vi "All-Indentify-To-Sort_Lite.vi"(6 "當前位置":i32, 7 "輸出顏色-位置":T1(array[cluster]), 8 "Error In":errorcluster, 11 "HiTechnicColorSensorV2 Ref In":cluster{"I2C Ref Out":T3}) -> (0 "Error Out":errorcluster, 2 "判斷結果":T2, 3 "HiTechnicColorSensorV2 Ref Out":cluster{"I2C Ref Out":T3}, 4 "離家數值":dbl[](array[numeric]), 5 "輸出顏色-位置 2":T1(array[cluster]))   [LabVIEW 2019]
uses:
  <vilib>/myRIO/Instrument Drivers/Onboard IO/I2C/typedefs/I2C Reference.ctl
  <vilib>/myRIO/Common/Instrument Driver Framework/Utilities/typedefs/myRIO Generic Hardware Reference.ctl
  <vilib>/myRIO/Common/Instrument Driver Framework/Utilities/typedefs/Hardware Version Enum.ctl
  <vilib>/myRIO/Common/Instrument Driver Framework/Utilities/typedefs/myRIO v1.0 Reference.ctl
  <vilib>/myRIO/Common/Instrument Driver Framework/Utilities/typedefs/Generic FPGA Reference.ctl
  <vilib>/myRIO/Common/Instrument Driver Framework/myRIO v1.0/I2C/typedefs/I2C Channels Enum.ctl
  <vilib>/myRIO/Instrument Drivers/Onboard IO/I2C/typedefs/I2C Configuration.ctl
  <vilib>/myRIO/Instrument Drivers/Onboard IO/I2C/typedefs/I2C Transfer Rate.ctl
  <vilib>/myRIO/Instrument Drivers/Onboard IO/I2C/I2C.lvlib
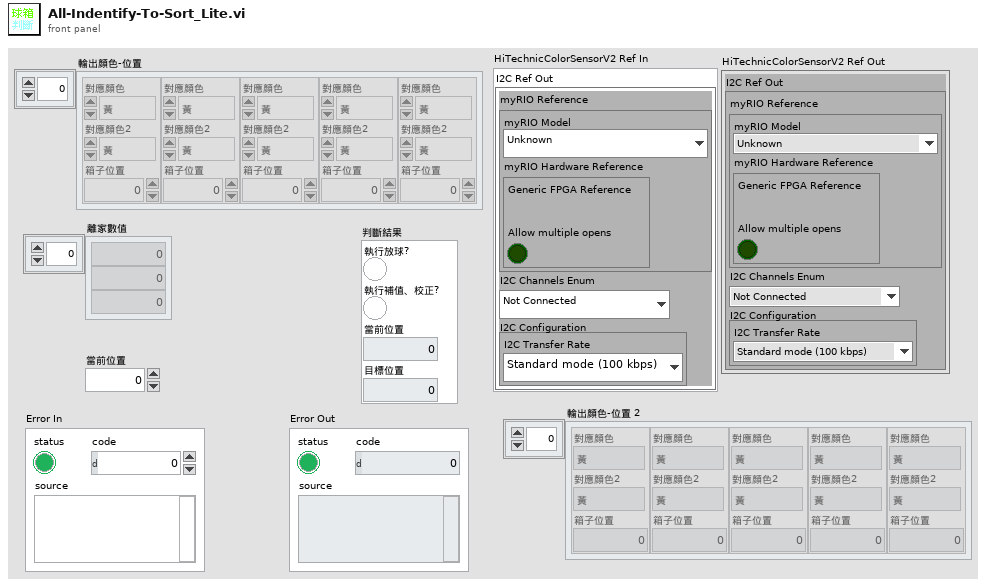
[diagram p1: front panel]
types:
  T1 = cluster{"對應顏色":enum16{"黃", "紅", "綠", "藍", "黑", "無"}, "對應顏色2":enum16{"黃", "紅", "綠", "藍", "黑", "無"}, "箱子位置":i32}[]
  T2 = cluster{"執行放球?":bool, "執行補值、校正?":bool, "當前位置":i32, "目標位置":i32}
  T3 = typedef "I2C.lvlib/I2C Reference.ctl" = cluster{"myRIO Reference":T4, "I2C Channels Enum":T8, "I2C Configuration":T9}
  T4 = typedef "myRIO Generic Hardware Reference.ctl" = cluster{"myRIO Model":T5, "myRIO Hardware Reference":T6}
  T5 = typedef "Hardware Version Enum.ctl" = enum16{"Unknown", "myRIO-1900", "myRIO-1950", "roboRIO", "NI ELVIS RIO CM", "ELVIS III"}
  T6 = typedef "myRIO v1.0 Reference.ctl" = cluster{"Generic FPGA Reference":T7, "Allow multiple opens":bool}
  T7 = typedef "Generic FPGA Reference.ctl" = refnum<k20>
  T8 = typedef "I2C Channels Enum.ctl" = enum16{"Not Connected", "A/I2C", "B/I2C", "I2C/I2C"}
  T9 = typedef "I2C.lvlib/I2C Configuration.ctl" = cluster{"I2C Transfer Rate":T10}
  T10 = typedef "I2C.lvlib/I2C Transfer Rate.ctl" = enum16{"Standard mode (100 kbps)", "Fast mode (400 kbps)"}
  T11 = cluster{"對應顏色":enum16{"黃", "紅", "綠", "藍", "黑", "無"}, "對應顏色2":enum16{"黃", "紅", "綠", "藍", "黑", "無"}, "箱子位置":i32}
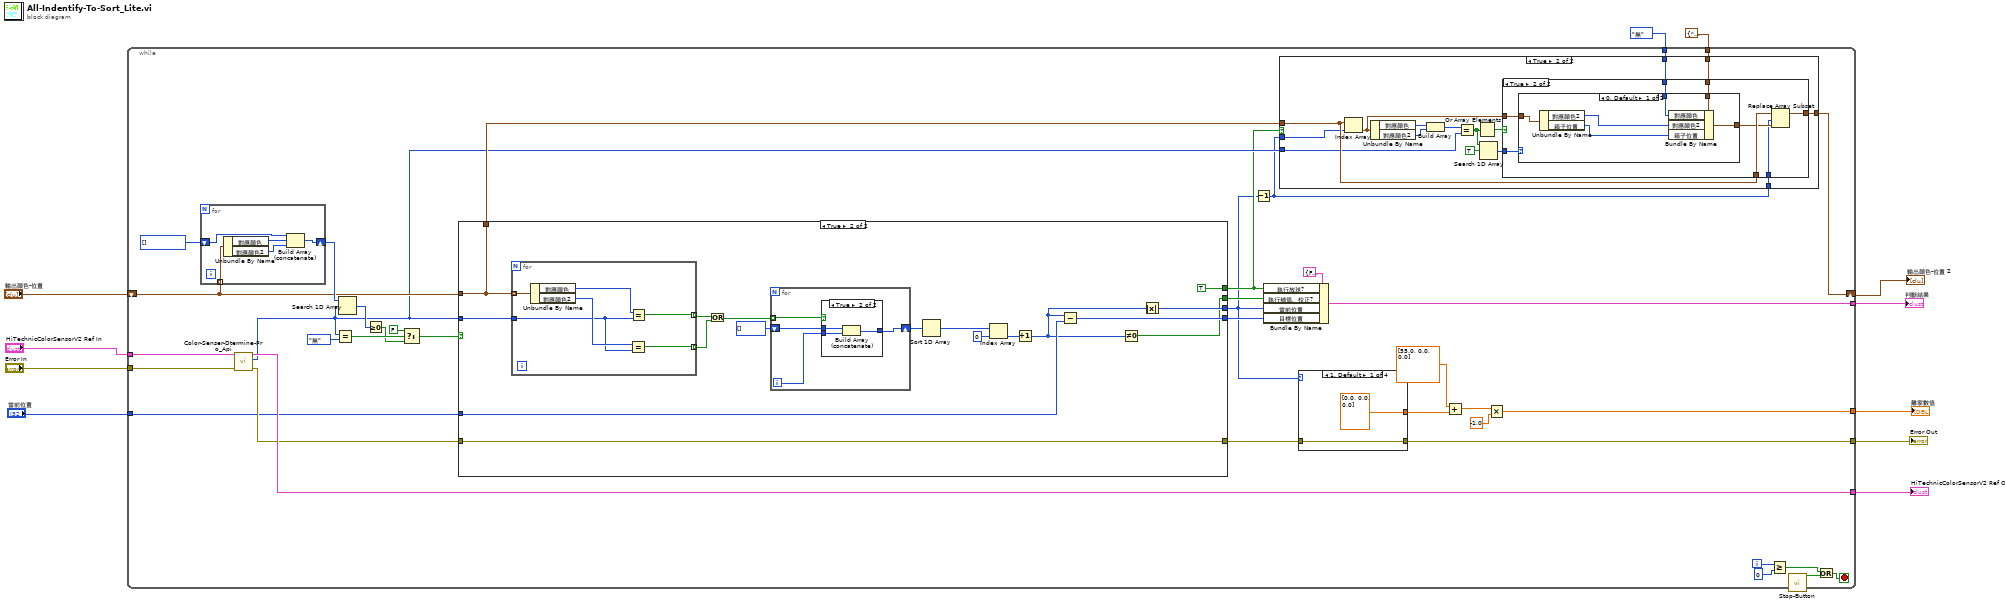
[diagram p0: block diagram]
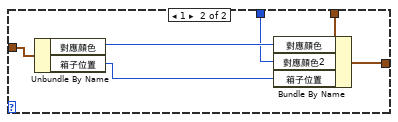
[diagram p4: hidden frame]
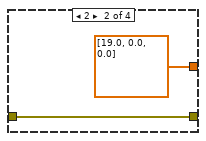
[diagram p5: hidden frame]
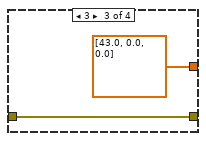
[diagram p6: hidden frame]
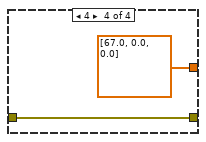
[diagram p7: hidden frame]
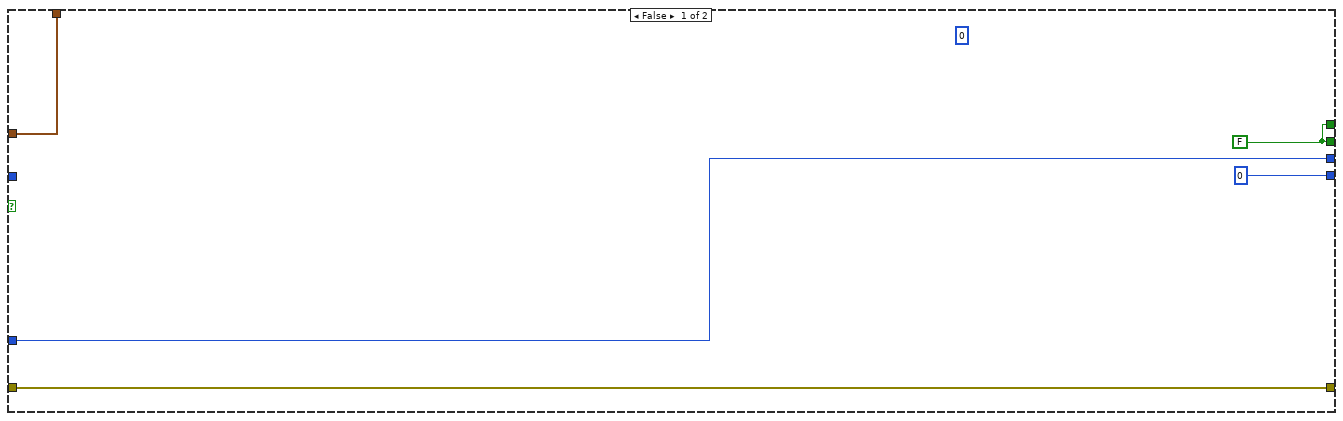
[diagram p8: hidden frame]
diagram:
  n1 = while {
    tunnel: "當前位置" -> [w21]
    tunnel: [w39] -> w7
    tunnel: [w35] -> w6
    shift-right: [w23] -> w4
    shift-left: "輸出顏色-位置" -> [w20]
    tunnel: "Error In" -> [w45]
    tunnel: [w29] -> w5
    tunnel: "HiTechnicColorSensorV2 Ref In" -> [w44]
    tunnel: [w43] -> w9
    tunnel: enum16{"黃", "紅", "綠", "藍", "黑", "無"}."無" ("對應顏色") -> [w18]
    tunnel: T11 {"對應顏色"=enum."黃", "對應顏色2"=enum."黃", "箱子位置"=0} ("element") -> [w17]
    i -> [w26]
    stop <- w28 stop-if-true
    w47 = enum16{"黃", "紅", "綠", "藍", "黑", "無"}[] [] items=["黃", "紅", "綠", "藍", "黑", "無"]
    n2 = for {
      tunnel: w20 -> [w99] mode=indexing
      shift-right: [w96] -> w46
      shift-left: w47 -> [w95]
      n3 = Unbundle By Name(w99) -> ("對應顏色"=w98:enum16{"黃", "紅", "綠", "藍", "黑", "無"}, "對應顏色2"=w97:enum16{"黃", "紅", "綠", "藍", "黑", "無"})
      n4 = Build Array (concatenate)(w95, w98, w97) -> (w96:enum16{"黃", "紅", "綠", "藍", "黑", "無"}[])
    }
    n5 = call "Color-Senser-Dtermine-Pro_Api.vi"("Error In"=w45, "HiTechnicColorSensorV2 Ref In"=w44) -> ("Error Out"=w31:errorcluster, "對應顏色"=w15:enum16{"黃", "紅", "綠", "藍", "黑", "無"}, "HiTechnicColorSensorV2 Ref Out"=w43:cluster{"I2C Ref Out":T3})  [unwired: 4 in, 3 out]
    n6 = Equal?(x=w15, y=enum16{"黃", "紅", "綠", "藍", "黑", "無"}."無") -> (x = y?=w34:bool)
    n7 = Search 1D Array(1D array=w46, element=w15) -> (index of element=w48:i32)  [unwired: 1 in]
    n8 = Greater Or Equal To 0?(x=w48) -> (x >= 0?=w32:bool)
    n9 = Select(t=FALSE, s=w34, f=w32) -> (s? t:f=w16:bool)
    n10 = case shown="True" w16 {
      tunnel: w20 -> [w100 w106]
      tunnel: [w104 w107] -> w36
      tunnel: [w104 TRUE ("放球校正?")] -> w14
      tunnel: [w103 w113] -> w12
      tunnel: w21 -> [w103 w114]
      tunnel: [0 w109] -> w22
      tunnel: w31 -> [w101 w112]
      tunnel: [w101 w112] -> w30
      tunnel: w15 -> [_ w111]
      tunnel: [w100 w106] -> w19
      frame False {
        (unwired) 0
        w104 = FALSE ("放球校正?")
      }
      frame True {
        n11 = for {
          tunnel: w106 -> [w135] mode=indexing
          tunnel: [w132] -> w121 mode=indexing
          tunnel: [w131] -> w120 mode=indexing
          tunnel: w111 -> [w130]
          n12 = Unbundle By Name(w135) -> ("對應顏色"=w134:enum16{"黃", "紅", "綠", "藍", "黑", "無"}, "對應顏色2"=w133:enum16{"黃", "紅", "綠", "藍", "黑", "無"})
          n13 = Equal?(x=w133, y=w130) -> (x = y?=w132:bool)
          n14 = Equal?(x=w134, y=w130) -> (x = y?=w131:bool)
        }
        n15 = Or(x=w120, y=w121) -> (x .or. y?=w119:bool[])
        n16 = for {
          tunnel: w119 -> [w125] mode=indexing
          shift-right: [w123] -> w117
          shift-left: i32[] [] -> [w122]
          i -> [w124]
          n17 = case shown="True" w125 {
            tunnel: w124 -> [_ w129]
            tunnel: [w126 w128] -> w123
            tunnel: w122 -> [w126 w127]
            frame False {
            }
            frame True {
              n18 = Build Array (concatenate)(w127, w129) -> (w128:i32[])
            }
          }
        }
        n19 = Sort 1D Array(array=w117) -> (sorted array=w115:i32[])
        n20 = Index Array(array=w115, index=0) -> (element=w105:i32)
        n21 = Increment(x=w105) -> (x+1=w108:i32)
        n22 = Subtract(x=w108, y=w114) -> (x-y=w109:i32)
        n23 = Not Equal To 0?(x=w108) -> (x != 0?=w107:bool)
        n24 = Absolute Value(x=w108) -> (abs(x)=w113:i32)
      }
    }
    n25 = Decrement(x=w12) -> (x-1=w13:i32)
    n26 = Bundle By Name(cluster=T2 {"執行放球?"=FALSE, "執行補值、校正?"=FALSE, "當前位置"=0, "目標位置"=0} ("input cluster"), "執行放球?"=w14, "執行補值、校正?"=w36, "當前位置"=w12, "目標位置"=w22) -> (w35:T2)
    n27 = case shown="True" w14 {
      tunnel: [w50 w57] -> w23
      tunnel: w19 -> [w50 w56]
      tunnel: w18 -> [_ w55]
      tunnel: w17 -> [_ w54]
      tunnel: w15 -> [_ w53]
      tunnel: w13 -> [_ w52]
      tunnel: w13 -> [_ w51]
      frame False {
      }
      frame True {
        n28 = Index Array(array=w56, index=w52) -> (element=w62:T11)
        n29 = Unbundle By Name(w62) -> ("對應顏色"=w65:enum16{"黃", "紅", "綠", "藍", "黑", "無"}, "對應顏色2"=w64:enum16{"黃", "紅", "綠", "藍", "黑", "無"})
        n30 = Build Array(w65, w64) -> (w63:enum16{"黃", "紅", "綠", "藍", "黑", "無"}[])
        n31 = Equal?(x=w63, y=w53) -> (x = y?=w60:bool[])
        n32 = Or Array Elements(Boolean array=w60) -> (logical OR=w61:bool)
        n33 = Search 1D Array(1D array=w60, element=TRUE) -> (index of element=w58:i32)  [unwired: 1 in]
        n34 = case shown="True" w61 {
          tunnel: w62 -> [_ w74]
          tunnel: w55 -> [_ w73]
          tunnel: w54 -> [_ w72]
          tunnel: w56 -> [w66 w71]
          tunnel: [w66 w69] -> w57
          tunnel: w58 -> [_ w68]
          tunnel: w51 -> [_ w67]
          frame False {
          }
          frame True {
            n35 = case shown="0, Default" w68 {
              tunnel: w74 -> [w80 w86]
              tunnel: w73 -> [w76 w83]
              tunnel: w72 -> [w79 w82]
              tunnel: [w75 w81] -> w70
              frame 0, Default {
                n36 = Unbundle By Name(w80) -> ("對應顏色2"=w78:enum16{"黃", "紅", "綠", "藍", "黑", "無"}, "箱子位置"=w77:i32)
                n37 = Bundle By Name(cluster=w79, "對應顏色"=w76, "對應顏色2"=w78, "箱子位置"=w77) -> (w75:T11)
              }
              frame 1 {
                n38 = Unbundle By Name(w86) -> ("對應顏色"=w85:enum16{"黃", "紅", "綠", "藍", "黑", "無"}, "箱子位置"=w84:i32)
                n39 = Bundle By Name(cluster=w82, "對應顏色"=w85, "對應顏色2"=w83, "箱子位置"=w84) -> (w81:T11)
              }
            }
            n40 = Replace Array Subset(array=w71, new element=w70, index=w67) -> (w69:T1)
          }
        }
      }
    }
    n41 = case shown="1, Default" w12 {
      tunnel: [dbl[] [0.0, 0.0, 0.0] dbl[] [19.0, 0.0, 0.0] dbl[] [43.0, 0.0, 0.0] dbl[] [67.0, 0.0, 0.0]] -> w42
      tunnel: w30 -> [w87 w89 w91 w93]
      tunnel: [w87 w89 w91 w93] -> w29
      frame 1, Default {
      }
      frame 2 {
      }
      frame 3 {
      }
      frame 4 {
      }
    }
    n42 = Add(x=dbl[] [55.0, 0.0, 0.0], y=w42) -> (x+y=w40:dbl[])
    n43 = Multiply(x=w40, y=-1.0) -> (x*y=w39:dbl[])
    n44 = Greater Or Equal?(x=w26, y=0) -> (x >= y?=w27:bool)
    n45 = call "Stop-Button.vi"() -> ("顯示按下?"=w24:bool)  [unwired: 10 in, 1 out]
    n46 = Or(x=w27, y=w24) -> (x .or. y?=w28:bool)
  }
  "Error Out" <- w5
  "HiTechnicColorSensorV2 Ref Out" <- w9
  "離家數值" <- w7
  "判斷結果" <- w6
  "輸出顏色-位置 2" <- w4
